vi "TEST GPR Graph X Control.vi"() -> ()   [LabVIEW 2011]
doc: "This VI Tests the GPR Graph XControl.\n\nAAL 9/09"
uses:
  XControl/GPR.xctl
panel:
  out "GPR":dbl[][](xcontrol)
  in  "File Path":path=path "C:/Exercises/Advanced Architectures in LabVIEW/Demonstrations/XControl/GPR Graph/Data/Real Data.asc"
  in  "Plot Type":u16(ring)=1 items=["Intensity Plot", "Wiggle Trace"]
  in  "Clear":bool
  in  "stop":bool
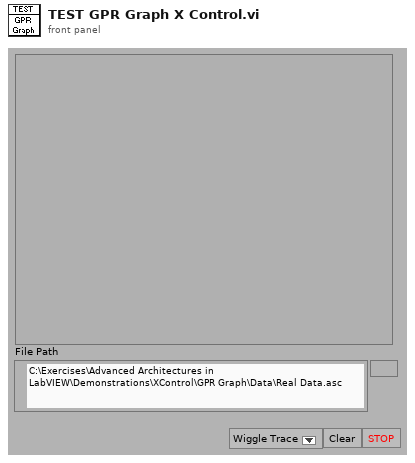
[diagram p1: front panel]
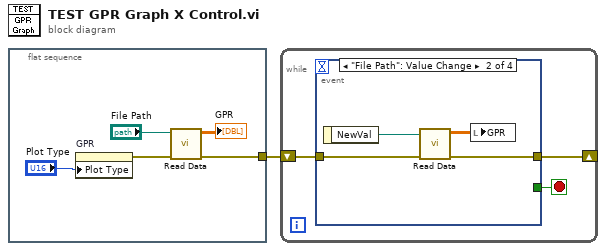
[diagram p0: block diagram]
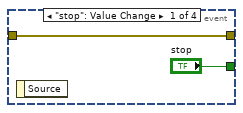
[diagram p2: hidden frame]
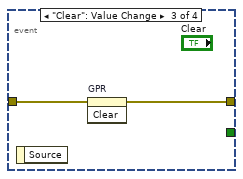
[diagram p3: hidden frame]
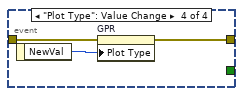
[diagram p4: hidden frame]
diagram:
  n1 = flat-sequence {
    tunnel: [w5] -> w1
    frame #0 {
      n2 = property on="GPR" class="GPR (strict)"("Plot Type"="Plot Type") -> (error out=w3:errorcluster)  [unwired: 2 in, 1 out]
      n3 = call "Read Data.vi"("error in"=w3, "file path"="File Path") -> ("error out"=w5:errorcluster, "Data"=→"GPR":dbl[][])  [unwired: 8 in]
    }
  }
  n4 = while {
    shift-right: [w8] -> _
    shift-left: w1 -> [w9]
    stop <- w7 stop-if-true
    n5 = event shown="[1] \"File Path\": Value Change" {
      selector: _ -> [_ _ _ _]
      dyn-events: _ -> [_ _ _ _]
      timeout: _ -> [_ _ _ _]
      tunnel: w9 -> [w11 w14 w17 w20]
      tunnel: [w11 w13 w16 w19] -> w8
      tunnel: ["stop" _ _ _] -> w7
      event "stop": Value Change {
        n6 = event-data() -> ()  [unwired: 1 in, 1 out]
      }
      event "File Path": Value Change {
        n7 = event-data() -> ("NewVal"=w15:path)  [unwired: 1 in]
        n8 = call "Read Data.vi"("error in"=w14, "file path"=w15) -> ("error out"=w13:errorcluster, "Data"=w12:dbl[][])  [unwired: 8 in]
        n9 = local write "GPR"(w12) -> ()
      }
      event "Clear": Value Change {
        n10 = event-data() -> ()  [unwired: 1 in, 1 out]
        n11 = invoke on="GPR" class="GPR (strict)" method="Clear"(error in=w17) -> (error out=w16:errorcluster)  [unwired: 2 in, 2 out]
      }
      event "Plot Type": Value Change {
        n12 = event-data() -> ("NewVal"=w18:u16)  [unwired: 1 in]
        n13 = property on="GPR" class="GPR (strict)"(error in=w20, "Plot Type"=w18) -> (error out=w19:errorcluster)  [unwired: 1 in, 1 out]
      }
    }
  }
